vi "lab session 2.1M.vi"(1 "Deg C":dbl) -> (0 "Deg F":dbl)   [LabVIEW 2020]
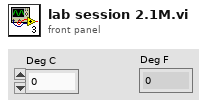
[diagram p1: front panel]
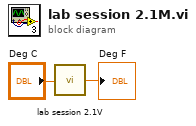
[diagram p0: block diagram]
diagram:
  n1 = call "lab session 2.1V.vi"("deg C"="Deg C") -> ("deg F"=→"Deg F":dbl)
